vi "libssh2_userauth_password.vi"(8 "error in (no error)":errorcluster, 9 "password":string, 10 "username":string, 11 "Session":T1) -> (0 "error out":errorcluster, 3 "return value":i32)   [LabVIEW 2013, in "libssh2.lvlib"]
uses:
  libssh2.lvlib
  Session Refnum.ctl
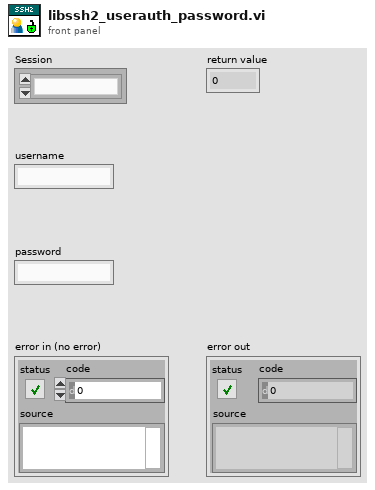
[diagram p1: front panel]
types:
  T1 = typedef "libssh2.lvlib/Session Refnum.ctl" = refnum<k1>
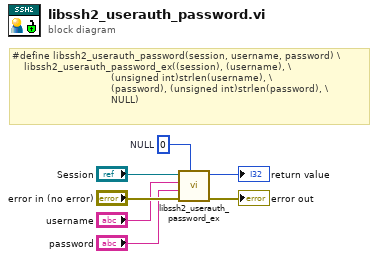
[diagram p0: block diagram]
diagram:
  w1 = u64 0  # NULL
  # "#define libssh2_userauth_password(session, username, password) \\\n    libssh2_userauth_password_ex((session), (username), \\\n                                 (unsigned int)strlen(username), \\\n                                 (password), (unsigned int)strlen(password), \\\n                                 NULL)"
  n1 = call "libssh2_userauth_password_ex.vi"("passwd_change_cb"=w1, "error in (no error)"="error in (no error)", "password"="password", "username"="username", "Session"="Session") -> ("error out"=→"error out":errorcluster, "return value"=→"return value":i32)  [unwired: 5 in]
